vi "TImeThresholdLogic(SubVI).vi"(2 "Position":dbl[](array[numeric]), 3 "Bits":dbl[](array[numeric]), 4 "Buffer":dbl[][](array[numeric])) -> (0 "Data":dbl[][](array[numeric]))   [LabVIEW 2017]
panel:
  out "출력 배열":dbl[][](array[numeric])
  out "부분배열":dbl[](array[numeric])
  out "x >= 0?":bool[](array[boolean])
  out "숫자":u32
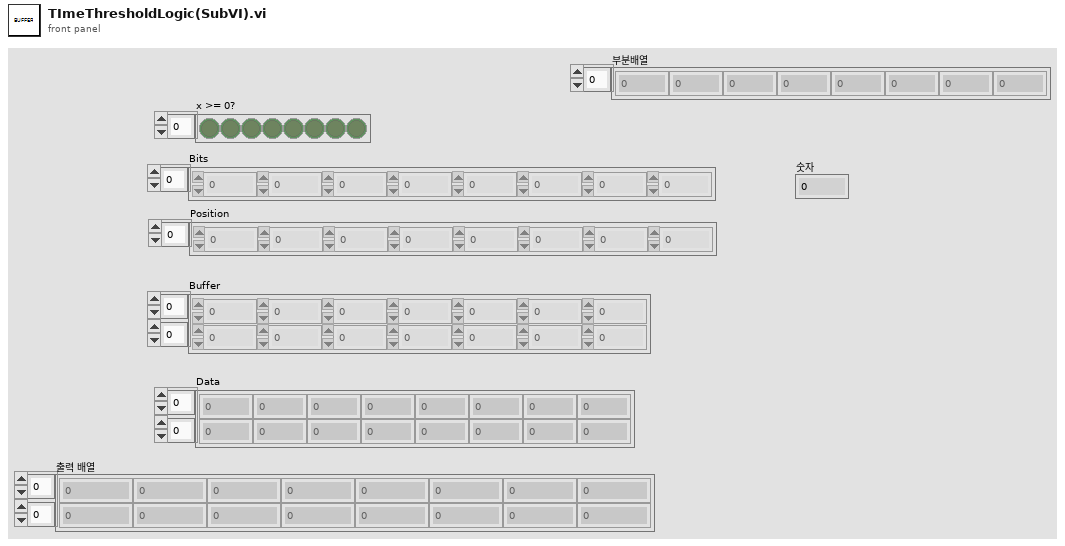
[diagram p1: front panel]
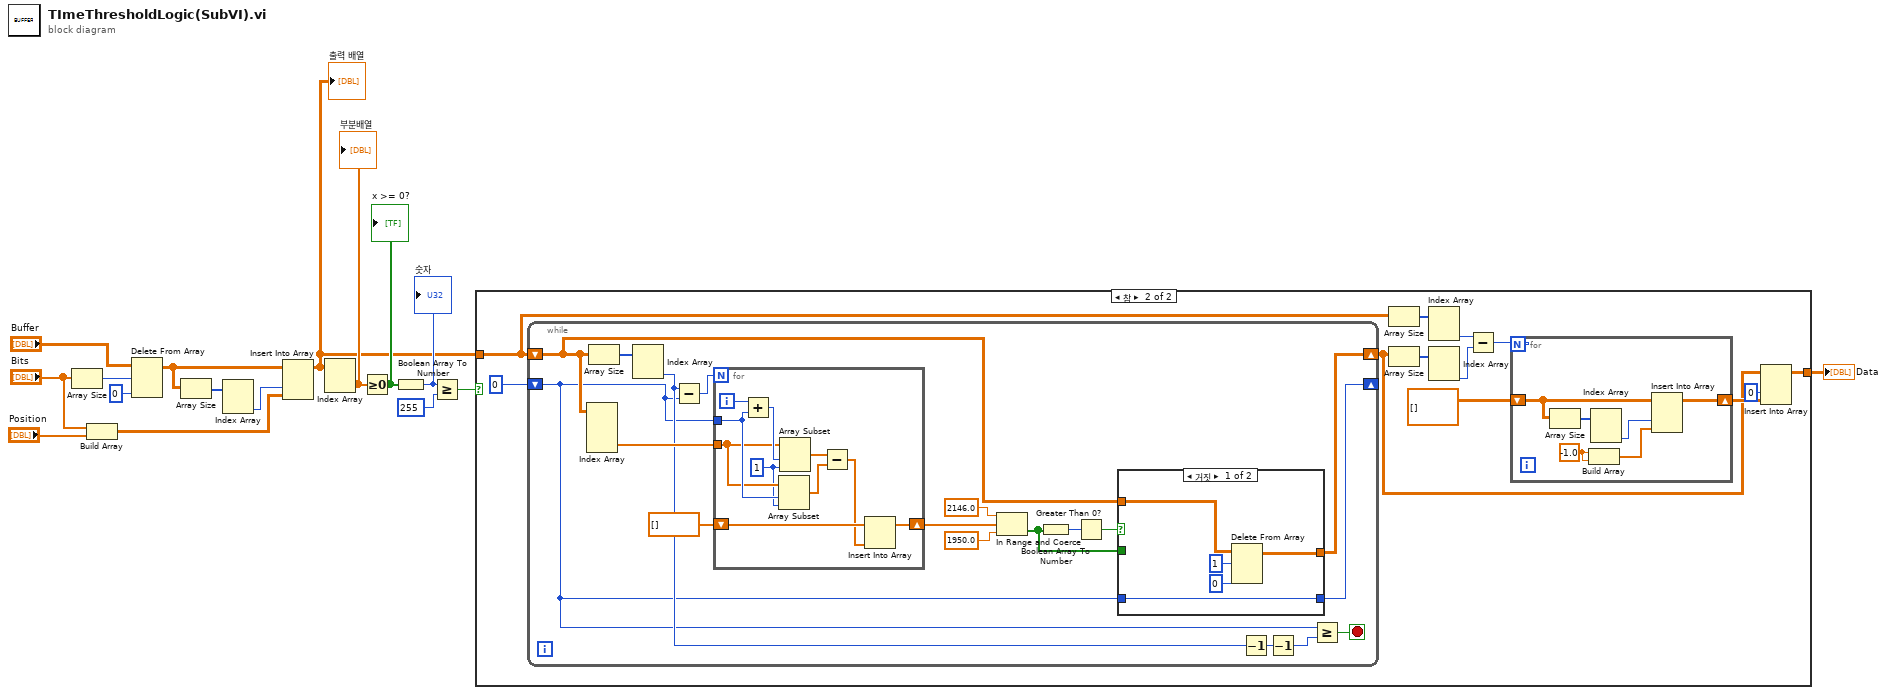
[diagram p0: block diagram]
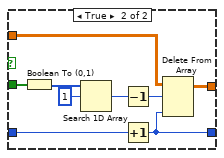
[diagram p3: hidden frame]
diagram:
  n1 = Array Size(array="Bits") -> (size(s)=w16:i32)
  n2 = Build Array("Bits", "Position") -> (w12:dbl[][])
  n3 = Delete From Array(array="Buffer", length=w16, index (col)=0 ("비활성화된 인덱스 (열)")) -> (array with subset deleted=w5:dbl[][])  [unwired: 1 in, 1 out]
  n4 = Array Size(array=w5) -> (size(s)=w11:i32[])
  n5 = Index Array(array=w11) -> (element #2=w10:i32)  [unwired: 2 in, 1 out]
  n6 = Insert Into Array(array=w5, index (col)=w10, new element=w12) -> (w4:dbl[][])  [unwired: 1 in]
  "출력 배열" <- w4
  n7 = Index Array(array=w4) -> (element=w9:dbl[])  [unwired: 2 in]
  "부분배열" <- w9
  n8 = Greater Or Equal To 0?(x=w9) -> (x >= 0?=w8:bool[])
  "x >= 0?" <- w8
  n9 = Boolean Array To Number(Boolean array=w8) -> (number=w7:u32)
  "숫자" <- w7
  n10 = Greater Or Equal?(x=w7, y=u32 255) -> (x >= y?=w3:bool)
  n11 = case shown="참" w3 {
    tunnel: w4 -> [w17 w28]
    tunnel: [w17 w18] -> w2
    frame False {
    }
    frame True {
      n12 = while {
        shift-right: [w43] -> _
        shift-left: 0 -> [w39]
        shift-right: [w38] -> w19
        shift-left: w28 -> [w42]
        stop <- w44 stop-if-true
        n13 = Index Array(array=w42) -> (element #2=w52:dbl[])  [unwired: 4 in, 1 out]
        n14 = Array Size(array=w42) -> (size(s)=w53:i32[])
        n15 = Index Array(array=w53) -> (element #2=w41:i32)  [unwired: 2 in, 1 out]
        n16 = Subtract(x=w41, y=w39) -> (x-y=w40:i32)
        n17 = for {
          N: w40 -> [_]
          tunnel: w52 -> [w74]
          tunnel: w39 -> [w75]
          shift-right: [w68] -> w46
          shift-left: dbl[] [] -> [w70]
          i -> [w77]
          w73 = 1 ("길이")
          n18 = Add(x=w77, y=w75) -> (x+y=w76:i32)
          n19 = Array Subset(array=w74, index=w75, length=w73) -> (w71:dbl[])
          n20 = Array Subset(array=w74, index=w76, length=w73) -> (w72:dbl[])
          n21 = Subtract(x=w72, y=w71) -> (x-y=w69:dbl[])
          n22 = Insert Into Array(array=w70, new element=w69) -> (w68:dbl[])  [unwired: 1 in]
        }
        n23 = In Range and Coerce(upper limit=2146.0 ("y"), x=w46, lower limit=1950.0 ("y")) -> (In Range?=w45:bool[])  [unwired: 1 out]
        n24 = Boolean Array To Number(Boolean array=w45) -> (number=w50:u32)
        n25 = Greater Than 0?(x=w50) -> (x > 0?=w49:bool)
        n26 = case shown="거짓" w49 {
          tunnel: w45 -> [_ w67]
          tunnel: w39 -> [w54 w63]
          tunnel: w42 -> [w58 w62]
          tunnel: [w55 w61] -> w38
          tunnel: [w54 w60] -> w43
          frame False {
            n27 = Delete From Array(array=w58, length=1 ("길이"), index (col)=0 ("비활성화된 인덱스 (열)")) -> (array with subset deleted=w55:dbl[][])  [unwired: 1 in, 1 out]
          }
          frame True {
            n28 = Boolean To (0,1)(Boolean=w67) -> (0, 1=w59:i16[])
            n29 = Search 1D Array(1D array=w59, element=i16 1 ("원소")) -> (index of element=w65:i32)  [unwired: 1 in]
            n30 = Decrement(x=w65) -> (x-1=w64:i32)
            n31 = Increment(x=w63) -> (x+1=w60:i32)
            n32 = Delete From Array(array=w62, length=w64, index (col)=w60) -> (array with subset deleted=w61:dbl[][])  [unwired: 1 in, 1 out]
          }
        }
        n33 = Decrement(x=w41) -> (x-1=w37:i32)
        n34 = Decrement(x=w37) -> (x-1=w36:i32)
        n35 = Greater Or Equal?(x=w39, y=w36) -> (x >= y?=w44:bool)
      }
      n36 = Array Size(array=w28) -> (size(s)=w27:i32[])
      n37 = Array Size(array=w19) -> (size(s)=w26:i32[])
      n38 = Index Array(array=w27) -> (element #2=w25:i32)  [unwired: 2 in, 1 out]
      n39 = Index Array(array=w26) -> (element #2=w24:i32)  [unwired: 2 in, 1 out]
      n40 = Subtract(x=w25, y=w24) -> (x-y=w23:i32)
      n41 = for {
        N: w23 -> [_]
        shift-right: [w30] -> w21
        shift-left: dbl[][] [] -> [w35]
        w32 = -1.0 ("원소")
        n42 = Array Size(array=w35) -> (size(s)=w34:i32[])
        n43 = Build Array(w32, w32) -> (w31:dbl[])
        n44 = Index Array(array=w34) -> (element #2=w33:i32)  [unwired: 2 in, 1 out]
        n45 = Insert Into Array(array=w35, index (col)=w33, new element=w31) -> (w30:dbl[][])  [unwired: 1 in]
      }
      n46 = Insert Into Array(array=w19, index (col)=0 ("비활성화된 인덱스 (열)"), new element=w21) -> (w18:dbl[][])  [unwired: 1 in]
    }
  }
  "Data" <- w2
